vi "to_json.vi"(8 "error in":errorcluster, 11 "mcapProtobufTimeseries in":refnum<class "mcapProtobufTimeseries.lvclass">) -> (0 "error out":errorcluster, 2 "json":string, 3 "mcapProtobufTimeseries out":refnum<class "mcapProtobufTimeseries.lvclass">, 4 "Not Default":bool)   [LabVIEW 2020, in "datasources.lvlib" / "mcapProtobufTimeseries.lvclass"]
uses:
  mcapProtobufTimeseries.lvclass
  C:/code/labview-client/lv_src/Nominal Client/datasources/datasource/datasource.lvclass
  datasource/datasource.lvclass/datasource.ctl
  mcapProtobufTimeseries.lvclass/mcapProtobufTimeseries.ctl
  7d555788-e1ce-4cf7-a60c-158276785de4.vi
  datasource/source.get.vi
  datasource/target.get.vi
  <vilib>/JDP Science/JSONtext/Variant to JSON Text.vi
  <vilib>/JDP Science/JSONtext/support/Format JSON Object.vi
  source/source.lvclass
  target/target.lvclass
  nominal types/channelFilter/channelFilter.lvclass
  <vilib>/JDP Science/JSONtext/LVClass Serializer/JSONtext LVClass Serializer.lvclass
  <vilib>/JDP Science/JSONtext/JSONtext.lvlib
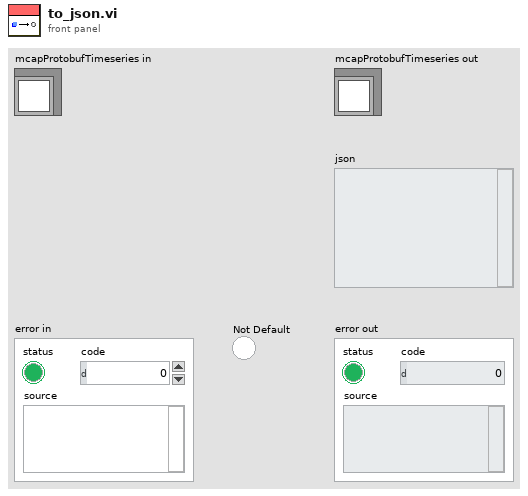
[diagram p1: front panel]
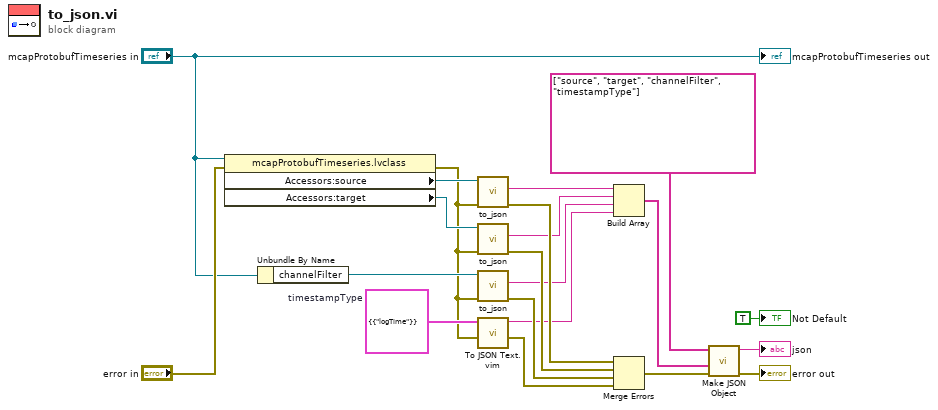
[diagram p0: block diagram]
diagram:
  w18 = cluster{"logTime":cluster{"type":string}} {"logTime"={"type"="logTime"}}  # timestampType
  n1 = property class="mcapProtobufTimeseries.lvclass"(reference="mcapProtobufTimeseries in", error in="error in") -> (error out=w12:errorcluster, "Accessors:source"=w21:refnum<class "source.lvclass">, "Accessors:target"=w20:refnum<class "target.lvclass">)  [unwired: 1 out]
  n2 = Unbundle By Name("mcapProtobufTimeseries in") -> ("channelFilter"=w19:refnum<class "channelFilter.lvclass">)
  n3 = call-dynamic "to_json.vi"("error in"=w12, "source in"=w21) -> ("error out"=w11:errorcluster, "json"=w16:string)  [unwired: 6 in, 2 out]
  n4 = call-dynamic "to_json.vi"("error in"=w12, "target in"=w20) -> ("error out"=w10:errorcluster, "json"=w4:string)  [unwired: 6 in, 2 out]
  n5 = call-dynamic "to_json.vi"("error in"=w12, "channelFilter in"=w19) -> ("error out"=w9:errorcluster, "json"=w3:string)  [unwired: 6 in, 2 out]
  n6 = call "To JSON Text.vim"("error in (no error)"=w12, "Anything"=w18) -> ("error out"=w8:errorcluster, "<JSON>"=w2:string)  [unwired: 8 in]
  n7 = Build Array(w16, w4, w3, w2) -> (w15:string[])
  n8 = Merge Errors(w11, w10, w9, w8) -> (w7:errorcluster)
  n9 = call <vilib>:"Make JSON Object.vi"("error in (no error)"=w7, "JSON Items"=w15, "Item Names"=string[] ["source", "target", "channelFilter", "timestampType"]) -> ("error out"=→"error out":errorcluster, "<JSON>"=→"json":string)  [unwired: 7 in]
  "mcapProtobufTimeseries out" <- "mcapProtobufTimeseries in"
  "Not Default" <- TRUE ("Not Default")
